vi "Asynchronous - Update BC to RT Data.vi"(5 "Raw Values (BC to RT)":T4, 7 "Map (BC to RT)":T1[](array[typedef]) {"Channel Data Reference" format="%.0x"}, 8 "Error (in)":errorcluster, 9 "Updated FIFO Index []":i32[](array[numeric]), 10 "U16 []":u16[](array[numeric])) -> (0 "Error (out)":errorcluster)   [LabVIEW 2020, in "Ballard MIL-1553 Engine.lvlib"]
uses:
  Ballard MIL-1553 Engine.lvlib
  Controls/RT Async_Raw Values.ctl
  Controls/RT Async_Raw Values to Messages Index_Association.ctl
  Controls/RT Async_Map BC2RT.ctl
  <vilib>/NI VeriStand/Custom Device API/Data Reference.ctl
  Controls/RT Async_Map_Type.ctl
  <userlib>/_OpenG.lib/array/array.llb/Remove Duplicates from 1D Array (I32)__ogtk.vi
  <instrlib>/BTI1553Lib/BTI1553LV.lvlib
  <vilib>/NI VeriStand/Custom Device API/Custom Device API.lvlib
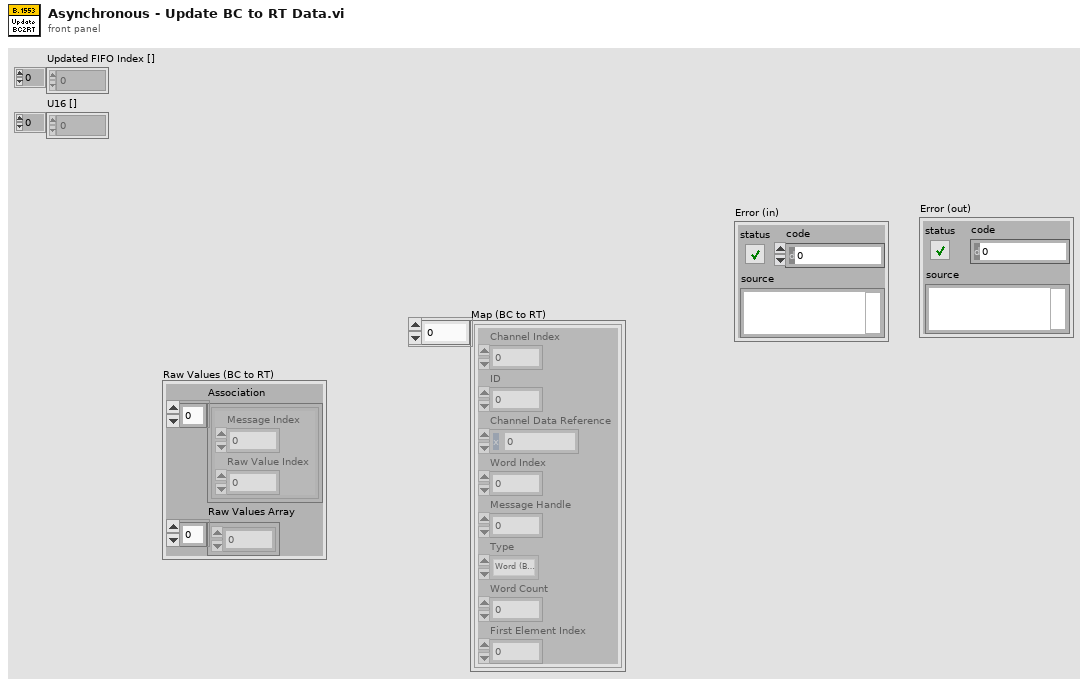
[diagram p1: front panel]
types:
  T1 = typedef "Ballard MIL-1553 Engine.lvlib/RT Async_Map BC2RT.ctl" = cluster{"Channel Index":i32, "ID":i32, "Channel Data Reference":T2, "Word Index":i32, "Message Handle":u64, "Type":T3, "Word Count":i32, "First Element Index":i32}
  T2 = typedef "Custom Device API.lvlib/Data Reference.ctl" = i32
  T3 = typedef "Ballard MIL-1553 Engine.lvlib/RT Async_Map_Type.ctl" = enum16{"Word (BC to RT)", "Word (MC (Rx))", "Acyclic Message Trigger", "Word (RT to ..)", "Word (RT to RT)", "Word (MC (Tx))", "RT Status", "BC Commands", "RT Commands"}
  T4 = typedef "Ballard MIL-1553 Engine.lvlib/RT Async_Raw Values.ctl" = cluster{"Association":T5[], "Raw Values Array":u16[]}
  T5 = typedef "Ballard MIL-1553 Engine.lvlib/RT Async_Raw Values to Messages Index_Association.ctl" = cluster{"Message Index":i32, "Raw Value Index":i32}
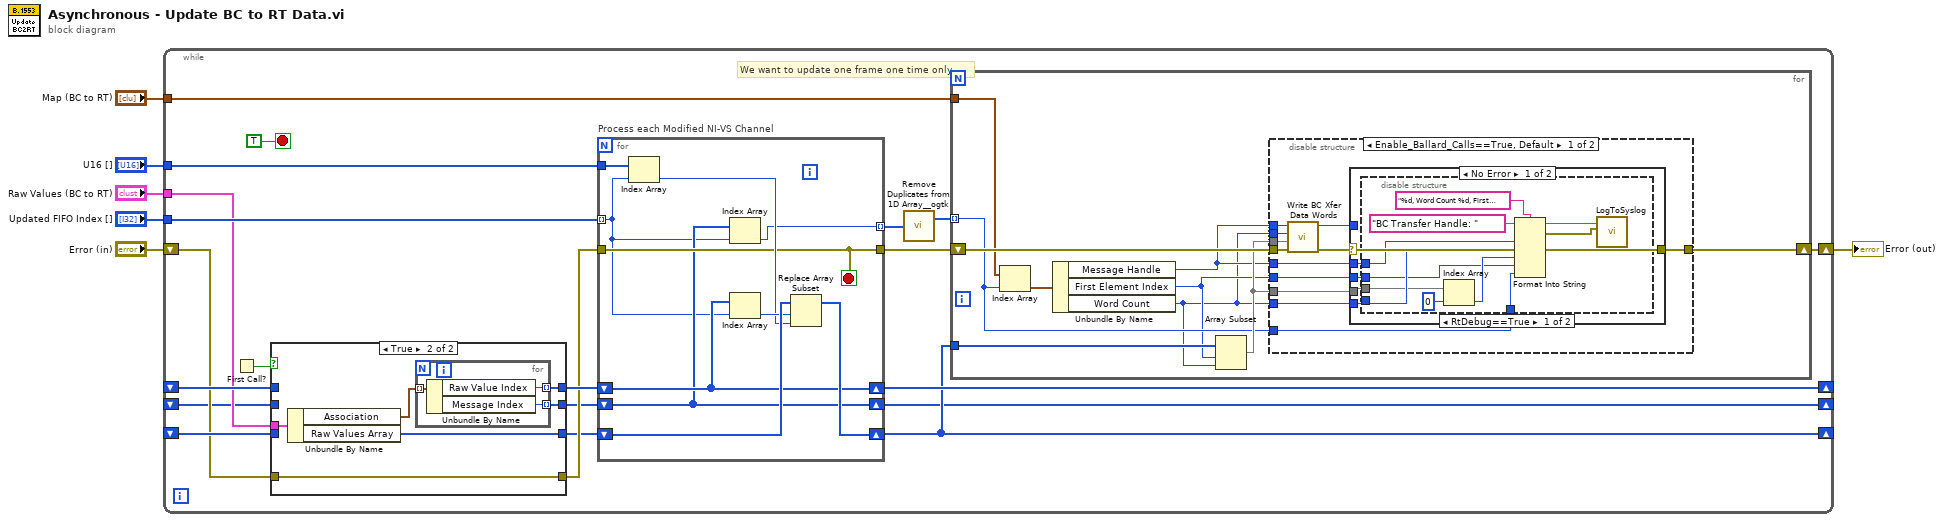
[diagram p0: block diagram]
diagram:
  n1 = while {
    tunnel: "Raw Values (BC to RT)" -> [w19]
    tunnel: "Updated FIFO Index []" -> [w27]
    tunnel: "U16 []" -> [w26]
    tunnel: "Map (BC to RT)" -> [w8]
    shift-right: [w15] -> w3
    shift-left: "Error (in)" -> [w18]
    shift-right: [w12] -> _
    shift-left: _ -> [w24]
    shift-right: [w22] -> _
    shift-left: _ -> [w21]
    shift-right: [w10] -> _
    shift-left: _ -> [w9]
    stop <- TRUE stop-if-true
    # "We want to update one frame one time only."
    n2 = First Call?() -> (First Call?: T/F=w20:bool)
    n3 = case shown="True" w20 {
      tunnel: w19 -> [_ w37]
      tunnel: [w31 w36] -> w7
      tunnel: w24 -> [w31 _]
      tunnel: [w30 w34] -> w23
      tunnel: w21 -> [w30 _]
      tunnel: w18 -> [w29 w32]
      tunnel: [w29 w32] -> w17
      tunnel: [w28 w33] -> w11
      tunnel: w9 -> [w28 _]
      frame False {
      }
      frame True {
        n4 = Unbundle By Name(w37) -> ("Association"=w35:T5[], "Raw Values Array"=w36:u16[])
        n5 = for {
          tunnel: w35 -> [w40] mode=indexing
          tunnel: [w39] -> w34 mode=indexing
          tunnel: [w38] -> w33 mode=indexing
          n6 = Unbundle By Name(w40) -> ("Raw Value Index"=w39:i32, "Message Index"=w38:i32)
        }
      }
    }
    n7 = for "Process each Modified NI-VS Channel" {
      tunnel: w27 -> [w42] mode=indexing
      tunnel: w26 -> [w50]
      tunnel: w17 -> [w44]
      tunnel: [w44] -> w16
      shift-right: [w48] -> w12
      shift-left: w7 -> [w49]
      shift-right: [w47] -> w22
      shift-left: w23 -> [w47]
      tunnel: [w41] -> w14 mode=indexing
      shift-right: [w43] -> w10
      shift-left: w11 -> [w43]
      stop <- w44 stop-if-true
      n8 = Index Array(array=w50, index=w42) -> (element=w45:u16)
      n9 = Index Array(array=w43, index=w42) -> (element=w41:i32)
      n10 = Index Array(array=w47, index=w42) -> (element=w46:i32)
      n11 = Replace Array Subset(array=w49, new element=w45, index=w46) -> (w48:u16[])
    }
    n12 = call-poly <userlib>:"Remove Duplicates from 1D Array__ogtk.vi"("Input Array"=w14) -> ("Output Array"=w13:i32[])  [unwired: 1 out]
    n13 = for {
      shift-right: [w59] -> w15
      shift-left: w16 -> [w60]
      tunnel: w13 -> [w55] mode=indexing
      tunnel: w12 -> [w58]
      tunnel: w8 -> [w54]
      n14 = Index Array(array=w54, index=w55) -> (element=w53:T1)
      n15 = Unbundle By Name(w53) -> ("Message Handle"=w56:u64, "First Element Index"=w52:i32, "Word Count"=w51:i32)
      n16 = Array Subset(array=w58, index=w52, length=w51) -> (w57:u16[])
      n17 = disable-structure shown="Enable_Ballard_Calls==True, Default" {
        disable-tunnel: w60 -> [w72 w91]
        disable-tunnel: [w69 w91] -> w59
        disable-tunnel: w56 -> [w64 _]
        disable-tunnel: w57 -> [w71 _]
        disable-tunnel: w57 -> [w67 _]
        disable-tunnel: w56 -> [w66 _]
        disable-tunnel: w55 -> [w65 _]
        disable-tunnel: w51 -> [w63 _]
        disable-tunnel: w52 -> [w62 _]
        disable-tunnel: w51 -> [w61 _]
        frame condition #0 (active) {
          n18 = call <instrlib>:"Write BC Xfer Data Words.vi"("error in (no error)"=w72, "data words"=w71, "data word count in"=w61, "bc transfer handle in"=w64) -> ("error out"=w70:errorcluster, "bc transfer handle out"=w68:u64)  [unwired: 5 in, 1 out]
          n19 = case shown="No Error" w70 {
            selector: w70 -> [w78 w90]
            tunnel: [w78 w90] -> w69
            tunnel: w68 -> [_ _]
            tunnel: w67 -> [w75 _]
            tunnel: w66 -> [w77 _]
            tunnel: w65 -> [w73 _]
            tunnel: w63 -> [w76 _]
            tunnel: w62 -> [w74 _]
            frame No Error {
              n20 = disable-structure shown="RtDebug==True" {
                disable-tunnel: w77 -> [w85 _]
                disable-tunnel: w76 -> [w84 _]
                disable-tunnel: w75 -> [w83 _]
                disable-tunnel: w74 -> [w80 _]
                disable-tunnel: w73 -> [w79 _]
                frame condition #0 (active) {
                  n21 = Index Array(array=w83, index=0) -> (element=w81:u16)
                  n22 = Format Into String(format string="%d, Word Count %d, First Value: %d, FE Index: %d, Message Index: %d.\\n", initial string="BC Transfer Handle: ", w85, w84, w81, w80, w79) -> (resulting string=w88:string, error out=w89:errorcluster)  [unwired: 1 in]
                  n23 = call "LogToSyslog.vi"("error in (no error)"=w89, "message"=w88) -> ()  [unwired: 8 in, 2 out]
                }
                frame condition #1 {
                }
              }
            }
            frame Error {
            }
          }
        }
        frame condition #1 {
        }
      }
    }
  }
  "Error (out)" <- w3
